vi "GSP_Logger_Global.vi"() -> ()   [LabVIEW 2015]
panel:
  out "Logger Online":bool
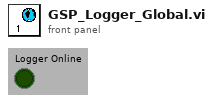
[diagram p1: front panel]
diagram:
